vi "Knob Scale and Name Updater.vi"(8 "error in":errorcluster, 11 "Cluster In":T1) -> (0 "error out":errorcluster, 3 "Cluster out":T1)   [LabVIEW 2018]
uses:
  Shared Controls/Range Updater.ctl
  Val Change Checker.vi
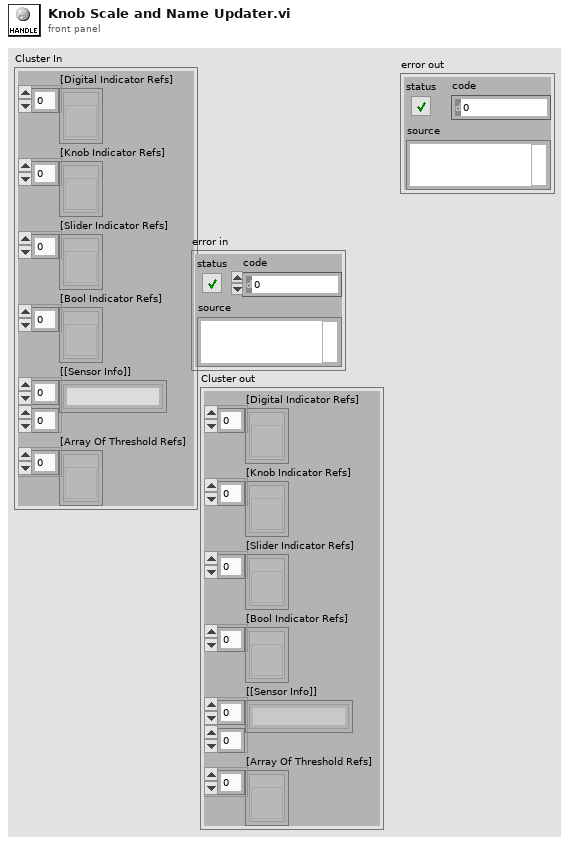
[diagram p1: front panel]
types:
  T1 = typedef "Range Updater.ctl" = cluster{"[Digital Indicator Refs]":refnum<vi>[], "[Knob Indicator Refs]":refnum<vi>[], "[Slider Indicator Refs]":refnum<vi>[], "[Bool Indicator Refs]":refnum<vi>[], "[[Sensor Info]]":string[][], "[Array Of Threshold Refs]":refnum<vi>[]}
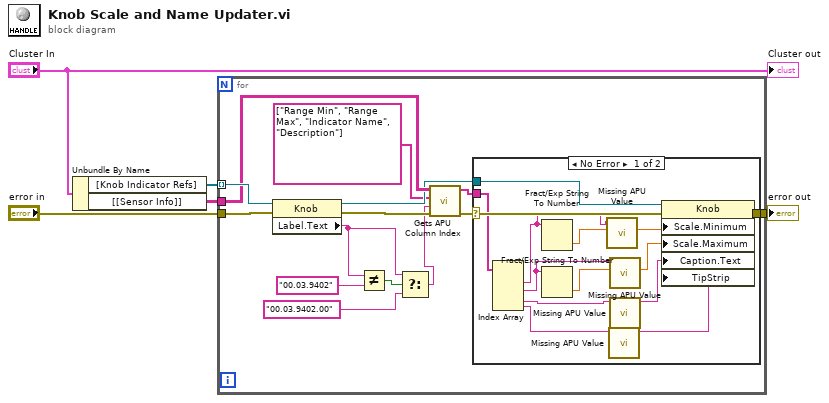
[diagram p0: block diagram]
diagram:
  n1 = Unbundle By Name("Cluster In") -> ("[Knob Indicator Refs]"=w4:refnum<vi>[], "[[Sensor Info]]"=w5:string[][])
  n2 = for {
    tunnel: w4 -> [w19] mode=indexing
    tunnel: "error in" -> [w18]
    tunnel: w5 -> [w16]
    tunnel: [w14] -> w2
    n3 = property class="Knob"(reference=w19, error in=w18) -> (reference out=w15:refnum<vi>, error out=w17:errorcluster, "Label.Text"=w7:string)
    n4 = Not Equal?(x=w7, y="00.03.9402") -> (x != y?=w9:bool)
    n5 = Select(t=w7, s=w9, f="00.03.9402.00" ("y")) -> (s? t:f=w6:string)
    n6 = call "Gets APU Column Index.vi"("error in (no error)"=w17, "Tag"=w6, "[Column Names]"=string[] ["Range Min", "Range Max", "Indicator Name", "Description"], "[[Array of Info]]"=w16) -> ("error out"=w13:errorcluster, "[Values out]"=w12:string[])  [unwired: 3 in, 3 out]
    n7 = case shown="No Error" w13 {
      selector: w13 -> [w33 w34]
      tunnel: [w32 w34] -> w14
      tunnel: w15 -> [w31 _]
      tunnel: w12 -> [w30 _]
      frame No Error {
        n8 = Index Array(array=w30) -> (element #1=w28:string, element #2=w26:string, element #3=w23:string, element #4=w21:string)  [unwired: 4 in]
        n9 = Fract/Exp String To Number(string=w28) -> (number=w29:dbl)  [unwired: 3 in, 1 out]
        n10 = Fract/Exp String To Number(string=w26) -> (number=w25:dbl)  [unwired: 3 in, 1 out]
        n11 = call "Missing APU Value.vi"("Num In"=w29, "String In"=w28) -> ("Num Out"=w27:dbl)  [unwired: 7 in, 2 out]
        n12 = call "Missing APU Value.vi"("String In"=w21) -> ("String Out"=w20:string)  [unwired: 8 in, 2 out]
        n13 = call "Missing APU Value.vi"("Num In"=w25, "String In"=w26) -> ("Num Out"=w24:dbl)  [unwired: 7 in, 2 out]
        n14 = call "Missing APU Value.vi"("String In"=w23) -> ("String Out"=w22:string)  [unwired: 8 in, 2 out]
        n15 = property class="Knob"(reference=w31, error in=w33, "Scale.Minimum"=w27, "Scale.Maximum"=w24, "Caption.Text"=w22, "TipStrip"=w20) -> (error out=w32:errorcluster)  [unwired: 1 out]
      }
      frame Error {
      }
    }
  }
  "error out" <- w2
  "Cluster out" <- "Cluster In"
